vi "Main Page.vi"(8 "error in (no error)":errorcluster, 11 "Node Ptr":T4 format="%.0x") -> (0 "error out":errorcluster)   [LabVIEW 2019, in "Diagnostics Addon System Explorer.lvlib"]
uses:
  Diagnostics Addon System Explorer.lvlib
  <vilib>/NI VeriStand/Custom Device API/Custom Device Item Ref.ctl
  Addon Shared/Types/Protocol.ctl
  Addon Shared/Types/Transport.ctl
  Types/FG.Action.ctl
  <vilib>/NI/NI VeriStand Hardware Resource Discovery/_Types/Filter Type.ctl
  Addon Shared/Types/986x.ctl
  Addon Shared/SubVIs/Constants.vi
  <vilib>/NI VeriStand/Custom Device API/NI VeriStand - Get Item Property.vi
  <vilib>/NI VeriStand/Custom Device API/Get Item Property (Boolean).vi
  <vilib>/NI VeriStand/Custom Device API/Get Item Property (String).vi
  <vilib>/NI VeriStand/Custom Device API/Get Item Property (Dependent File).vi
  <vilib>/NI VeriStand/Custom Device API/Get Item Property (Variant).vi
  <vilib>/NI VeriStand/Custom Device API/Get Item Property (U32).vi
  <vilib>/NI/NI VeriStand Advanced SysDef API/SysDef API/SysDef.Property.Set.vi
  <vilib>/NI/NI VeriStand Advanced SysDef API/_SubVIs/SysDef.Property.Set.String.vi
  <vilib>/NI/NI VeriStand Advanced SysDef API/_SubVIs/SysDef.Property.Set.Variant.vi
  <vilib>/NI/NI VeriStand Advanced SysDef API/_SubVIs/SysDef.Property.Set.U32.vi
  <vilib>/NI/NI VeriStand Advanced SysDef API/_SubVIs/SysDef.Property.Set.Boolean.vi
  <vilib>/NI VeriStand/Custom Device API/Custom Device API.lvlib
  Addon Shared/Diagnostics Addon Shared.lvlib
  <vilib>/NI/NI VeriStand Hardware Resource Discovery/NIVS Hardware Discovery.lvlib
panel:
  in  "Tab Control":T1(tab)
  in  "CAN Browse":bool
  out "Version":string
  in  "Termination":bool
  in  "Name":string
  in  "Description":string
  out "Diagnostic Protocol":T2
  in  "Port":string
  in  "Baud Rate":u64=250000
  in  "Enable Stream":bool
  in  "FD Baud Rate":u64=250000
  in  "Max DLC":u16
  in  "IO Mode":u32(ring) items=["CAN 2.0", "CAN FD", "CAN FD+BRS"]
  in  "Timeout":u32 caption="Comm Timeout (ms)"
  in  "Fill Byte":u8=255 format="%.0x"
  in  "Fill Frame":bool
  in  "Transport Protocol":T3
  in  "VW TP Channel ID":u32 format="%.0x"
  in  "Receive UUDT ID":u32 format="%.0x"
  in  "Receive Extension":u8 format="%.0x"
  in  "Receive ID":u32 format="%.0x"
  in  "Transmit Extension":u8 format="%.0x"
  in  "Transmit ID":u32 format="%.0x"
  in  "NAD":u8
  in  "LIN Cluster":refnum<k21>
  in  "RIO Browse":bool
  in  "RIO Device":string
  in  "Enable Bitfile":bool
  in  "Bitfile Path":path
  in  "Header":cluster{"Section Name":string}={"Section Name"="Custom Device Item Settings"}
  in  "SHDocVw.IWebBrowser":refnum<k7>(container)
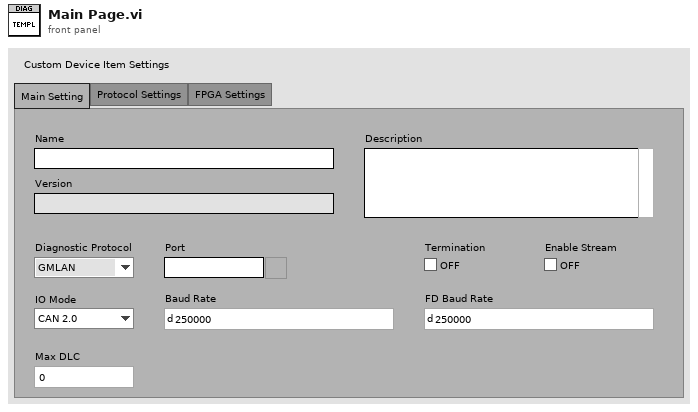
[diagram p1: front panel]
types:
  T1 = enum32{"Main Setting", "Protocol Settings", "FPGA Settings"}
  T2 = typedef "Diagnostics Addon Shared.lvlib/Protocol.ctl" = enum16{"GMLAN", "KWP-2000", "UDS", "User-Defined"}
  T3 = typedef "Diagnostics Addon Shared.lvlib/Transport.ctl" = enum16{"ISO TP - Normal Mode", "ISO TP - Mixed Mode", "VW TP 2.0", "Diagnostics on IP", "ISO TP LIN"}
  T4 = typedef "Custom Device API.lvlib/Custom Device Item Ref.ctl" = u64
  T5 = typedef "Diagnostics Addon System Explorer.lvlib/FG.Action.ctl" = enum16{"Get", "Set"}
  T6 = typedef "Custom Device API.lvlib/Custom Device Item Info.ctl" = cluster{"Name":string, "Is Channel":bool, "GUID":string, "Is Waveform":bool}
  T7 = typedef "Diagnostics Addon Shared.lvlib/986x.ctl" = cluster{"Enable":bool, "RIO Device":string, "Bitfile":path}
  T8 = typedef "Diagnostics Addon Shared.lvlib/CAN.ctl" = cluster{"Interface":T9, "Baud Rate":u64, "Diagnostic Protocol":T2, "Transport Protocol":T3, "Transmit ID":u32, "Receive ID":u32, "Transmit Extension":u8, "Receive Extension":u8, "Receive UUDT ID":u32, "Enable Stream":bool, "VW TP Channel ID":u32, "Fill Frame":bool, "Fill Byte":u8, "Termination":bool, "LIN Cluster":refnum<k21>, "NAD":u8, "IO Mode":u32, "Max DLC":u16, "FD Baud Rate":u64, "Timeout":u32}
  T9 = typedef "Diagnostics Addon Shared.lvlib/CAN.Interface.ctl" = string
  T10 = typedef "NIVS Hardware Discovery.lvlib/Filter Type.ctl" = enum16{"Device Category", "Product Name", "Ethernet", "XNET", "VISA", "FPGA", "EtherCAT Master", "DAQmx", "GPIB", "Serial"}
  T11 = typedef "Custom Device API.lvlib/Custom Device Commands.ctl" = enum16{"Default", "Item renamed", "Shutdown", "Dynamic button pressed"}
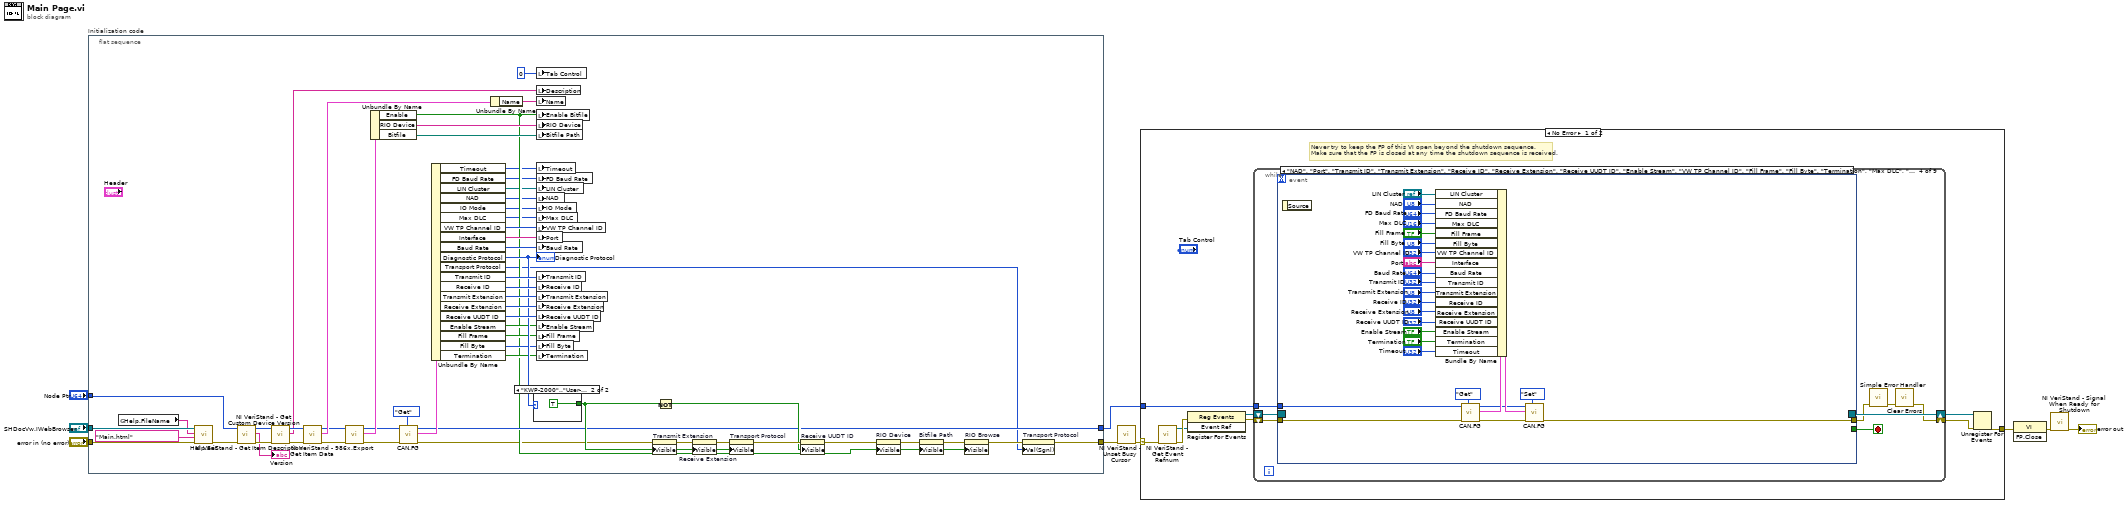
[diagram p0: block diagram]
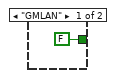
[diagram p2: hidden frame]
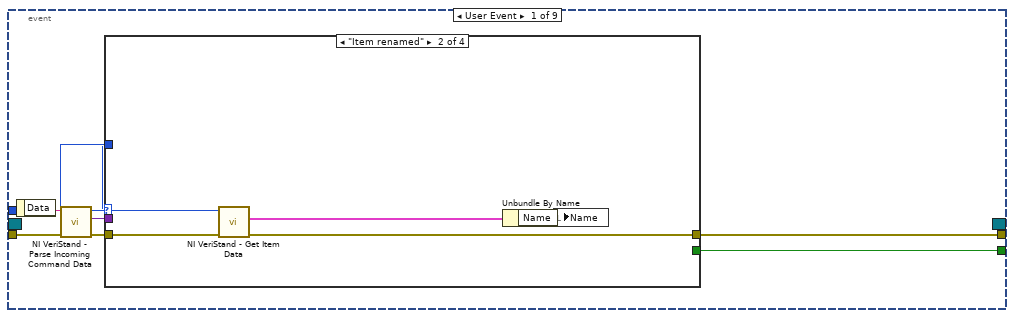
[diagram p3: hidden frame]
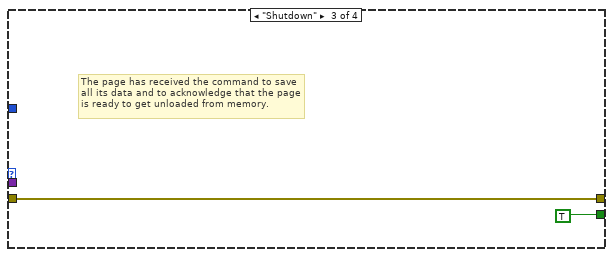
[diagram p5: hidden frame]
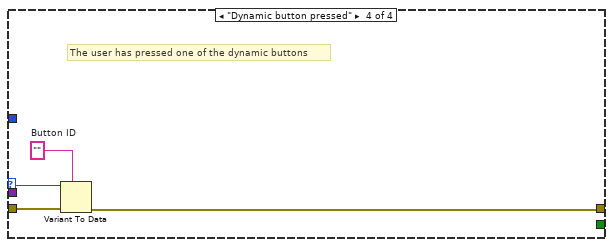
[diagram p6: hidden frame]
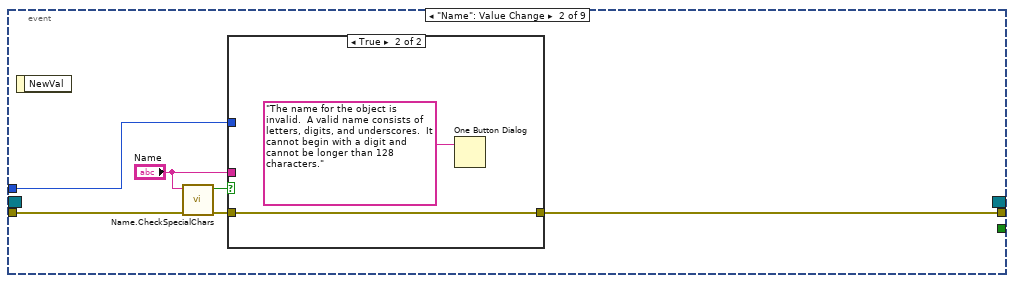
[diagram p7: hidden frame]
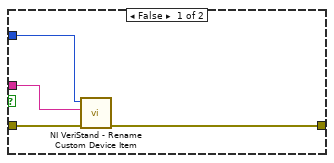
[diagram p8: hidden frame]
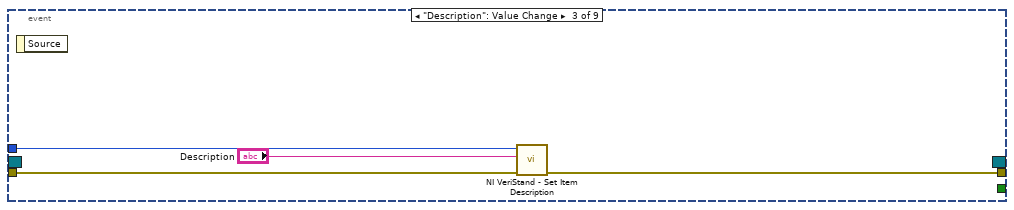
[diagram p9: hidden frame]
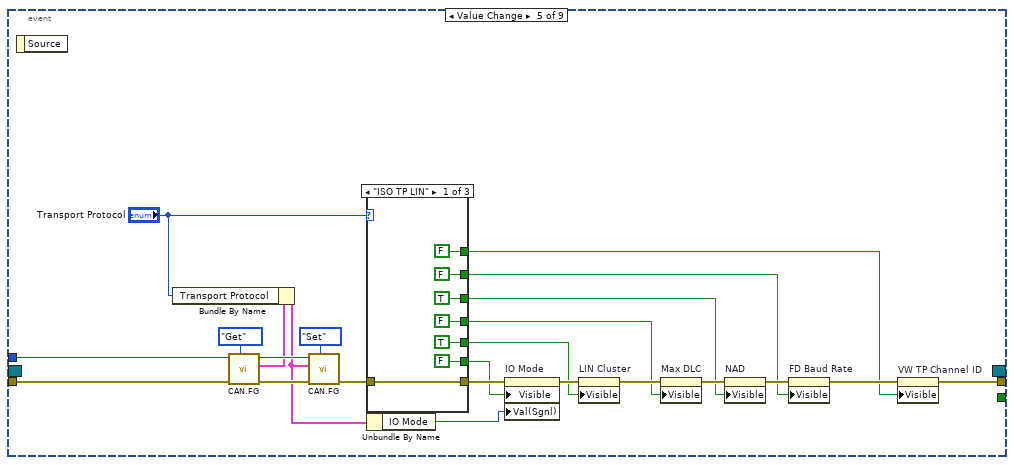
[diagram p10: hidden frame]
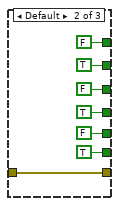
[diagram p11: hidden frame]
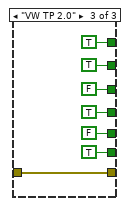
[diagram p12: hidden frame]
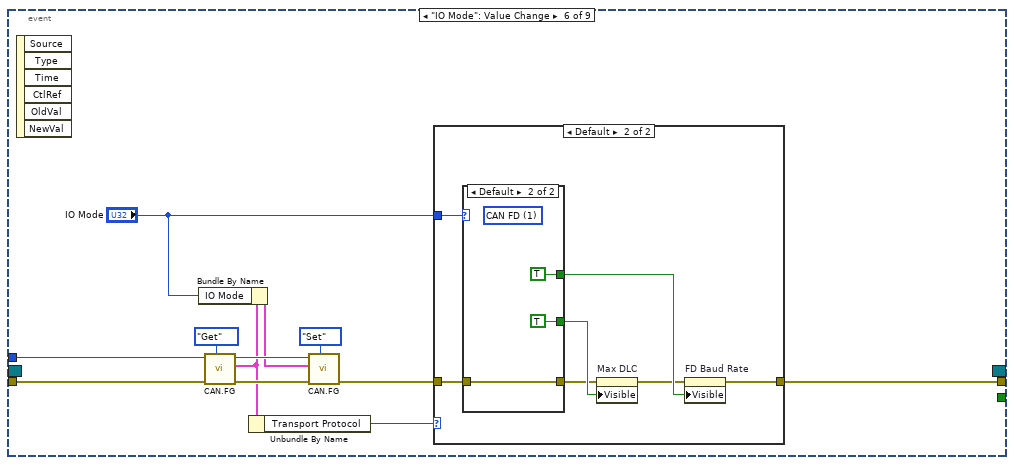
[diagram p13: hidden frame]
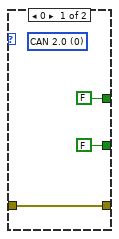
[diagram p15: hidden frame]
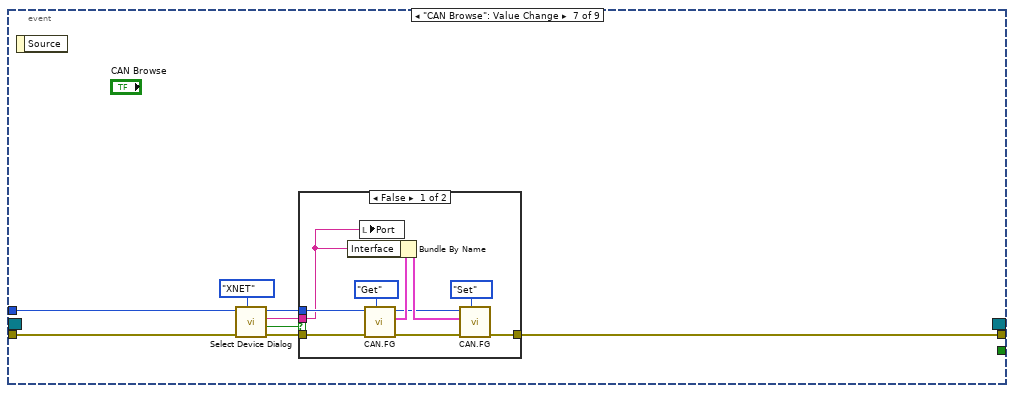
[diagram p16: hidden frame]
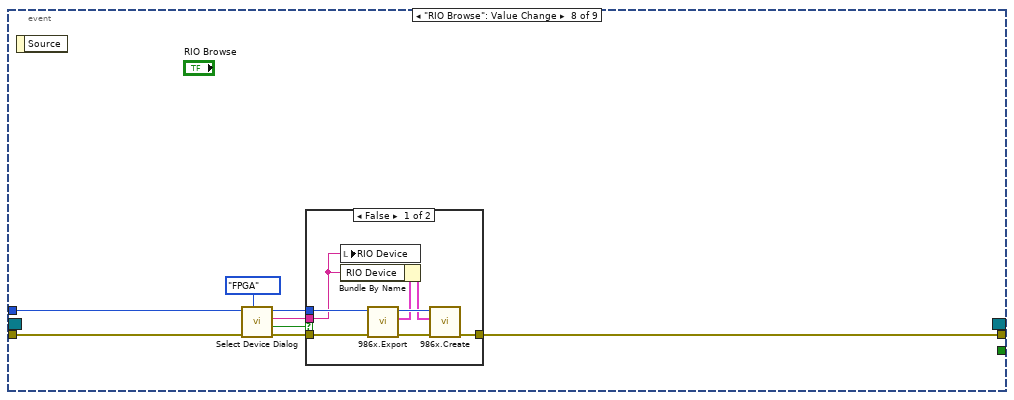
[diagram p18: hidden frame]
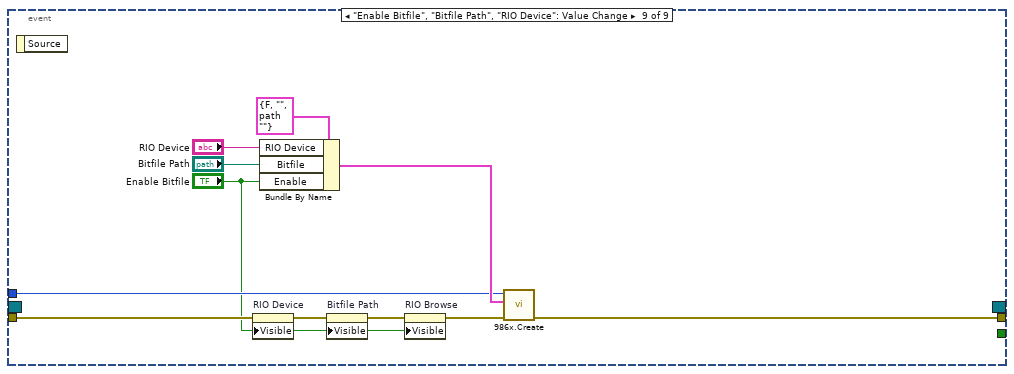
[diagram p20: hidden frame]
diagram:
  n1 = flat-sequence "Initialization code" {
    tunnel: "error in (no error)" -> [w61]
    tunnel: "Node Ptr" -> [w28]
    tunnel: [w11] -> w5
    tunnel: [w30] -> w2
    tunnel: "SHDocVw.IWebBrowser" -> [w60]
    frame #0 {
      n2 = global read "Constants.vi" "Help.FileName"() -> (w10:string)
      n3 = call "Help.Set.vi"("error in (no error)"=w61, "HTML File"="Main.html", "Main CHM File"=w10, "SHDocVw.IWebBrowser2"=w60) -> ("error out"=w29:errorcluster)  [unwired: 7 in]
      n4 = call <vilib>:"NI VeriStand - Get Custom Device Version.vi"("error in (no error)"=w29, "Device Ref in"=w28) -> ("error out"=w26:errorcluster, "Value"=→"Version":string, "Device Ref out"=w27:T4)  [unwired: 7 in]
      n5 = call <vilib>:"NI VeriStand - Get Item Description.vi"("error in (no error)"=w26, "Item Ref in"=w27) -> ("error out"=w64:errorcluster, "Description"=w65:string, "Item Ref out"=w66:T4)  [unwired: 7 out]
      n6 = call <vilib>:"NI VeriStand - Get Item Data.vi"("error in (no error)"=w64, "Item Ref in"=w66) -> ("error out"=w36:errorcluster, "Item Info"=w63:T6, "Item Ref out"=w35:T4)  [unwired: 7 out]
      n7 = call "986x.Export.vi"("error in (no error)"=w36, "Device Item Ref in"=w35) -> ("error out"=w34:errorcluster, "986x Support"=w37:T7, "Item Ref out"=w33:T4)  [unwired: 7 in]
      n8 = Unbundle By Name(w37) -> ("Enable"=w21:bool, "RIO Device"=w31:string, "Bitfile"=w32:path)
      n9 = call "CAN.FG.vi"("Action"=FG.Action."Get", "error in (no error)"=w34, "Device Item Ref in"=w33) -> ("error out"=w13:errorcluster, "Diagnostics Basic Configuration"=w58:T8, "Device Item Ref out"=w30:T4)  [unwired: 6 in]
      n10 = Unbundle By Name(w58) -> ("Timeout"=w12:u32, "FD Baud Rate"=w20:u64, "LIN Cluster"=w16:refnum<k21>, "NAD"=w19:u8, "IO Mode"=w14:u32, "Max DLC"=w18:u16, "VW TP Channel ID"=w44:u32, "Interface"=w57:T9, "Baud Rate"=w56:u64, "Diagnostic Protocol"=w50:T2, "Transport Protocol"=w15:T3, "Transmit ID"=w55:u32, "Receive ID"=w54:u32, "Transmit Extension"=w53:u8, "Receive Extension"=w51:u8, "Receive UUDT ID"=w52:u32, "Enable Stream"=w45:bool, "Fill Frame"=w39:bool, "Fill Byte"=w40:u8, "Termination"=w38:bool)
      "Diagnostic Protocol" <- w50
      n11 = Unbundle By Name(w63) -> ("Name"=w62:string)
      n12 = case shown="\"KWP-2000\"..\"User-Defined\"" w50 {
        tunnel: [FALSE TRUE] -> w42
        frame "GMLAN" {
        }
        frame "KWP-2000".."User-Defined" {
        }
      }
      n13 = local write "Tab Control"(0) -> ()
      n14 = local write "Description"(w65) -> ()
      n15 = local write "Name"(w62) -> ()
      n16 = local write "Enable Bitfile"(w21) -> ()
      n17 = local write "RIO Device"(w31) -> ()
      n18 = local write "Bitfile Path"(w32) -> ()
      n19 = local write "Timeout"(w12) -> ()
      n20 = local write "FD Baud Rate"(w20) -> ()
      n21 = local write "LIN Cluster"(w16) -> ()
      n22 = local write "NAD"(w19) -> ()
      n23 = local write "IO Mode"(w14) -> ()
      n24 = local write "Max DLC"(w18) -> ()
      n25 = local write "VW TP Channel ID"(w44) -> ()
      n26 = local write "Port"(w57) -> ()
      n27 = local write "Baud Rate"(w56) -> ()
      n28 = local write "Transmit ID"(w55) -> ()
      n29 = local write "Receive ID"(w54) -> ()
      n30 = local write "Transmit Extension"(w53) -> ()
      n31 = local write "Receive Extension"(w51) -> ()
      n32 = local write "Receive UUDT ID"(w52) -> ()
      n33 = local write "Enable Stream"(w45) -> ()
      n34 = local write "Fill Frame"(w39) -> ()
      n35 = local write "Fill Byte"(w40) -> ()
      n36 = local write "Termination"(w38) -> ()
      n37 = property on="Transmit Extension" class="DigNum (strict)"(error in=w13, "Visible"=w42) -> (error out=w49:errorcluster)  [unwired: 1 in, 1 out]
      n38 = Not(x=w42) -> (.not. x?=w46:bool)
      n39 = property on="Receive Extension" class="DigNum (strict)"(error in=w49, "Visible"=w42) -> (error out=w48:errorcluster)  [unwired: 1 in, 1 out]
      n40 = property on="Transport Protocol" class="Enum (strict)"(error in=w48, "Visible"=w42) -> (error out=w47:errorcluster)  [unwired: 1 in, 1 out]
      n41 = property on="Receive UUDT ID" class="DigNum (strict)"(error in=w47, "Visible"=w46) -> (error out=w22:errorcluster)  [unwired: 1 in, 1 out]
      n42 = property on="RIO Device" class="Str"(error in=w22, "Visible"=w21) -> (error out=w24:errorcluster)  [unwired: 1 in, 1 out]
      n43 = property on="Bitfile Path" class="Path"(error in=w24, "Visible"=w21) -> (error out=w23:errorcluster)  [unwired: 1 in, 1 out]
      n44 = property on="RIO Browse" class="Bool"(error in=w23, "Visible"=w21) -> (error out=w17:errorcluster)  [unwired: 1 in, 1 out]
      n45 = property on="Transport Protocol" class="Enum (strict)"(error in=w17, "Val(Sgnl)"=w15) -> (error out=w11:errorcluster)  [unwired: 1 in, 1 out]
    }
  }
  n46 = call <vilib>:"NI VeriStand - Unset Busy Cursor.vi"("error in (no error)"=w5) -> ("error out"=w4:errorcluster)  [unwired: 10 out]
  n47 = case shown="No Error" w4 {
    selector: w4 -> [w69 w268]
    tunnel: [w74 w266] -> w9
    tunnel: w2 -> [w70 _]
    frame No Error {
      # "Never try to keep the FP of this VI open beyond the shutdown sequence.\nMake sure that the FP is closed at any time the shutdown sequence is received."
      n48 = call <vilib>:"NI VeriStand - Get Event Refnum.vi"("error in (no error)"=w69) -> ("error out"=w77:errorcluster, "Event Ref"=w73:refnum<user-event>)  [unwired: 9 out]
      n49 = register-events(error in=w77, w73) -> (reference out=w71:refnum<event-registration>, error out=w72:errorcluster)  [unwired: 1 in]
      n50 = while {
        tunnel: w70 -> [w81]
        shift-right: [w78] -> w75
        shift-left: w72 -> [w84]
        shift-right: [w85] -> w76
        shift-left: w71 -> [w83]
        stop <- w82 stop-if-true
        n51 = event shown="[3] \"NAD\", \"Port\", \"Transmit ID\", \"Transmit Extension\", \"Receive ID\", \"Receive Extension\", \"Receive UUDT ID\", \"Enable Stream\", \"VW TP Channel ID\", \"Fill Frame\", \"Fill Byte\", \"Termination\", \"Max DLC\", \"FD Baud Rate\", \"LIN Cluster\", \"Baud Rate\", \"Timeout\": Value Change" {
          selector: w83 -> [_ _ _ _ _ _ _ _ _]
          dyn-events: [_ _ _ _ _ _ _ _ _] -> w85
          timeout: _ -> [_ _ _ _ _ _ _ _ _]
          tunnel: w84 -> [w93 w108 w120 w147 w171 w204 w225 w243 w260]
          tunnel: [w89 _ _ _ _ _ _ _ _] -> w82
          tunnel: [w88 w111 w119 w131 w149 w196 w226 w245 w262] -> w80
          tunnel: w81 -> [w87 w110 w121 w146 w170 w203 w224 w241 w261]
          event User Event {
            n52 = event-data() -> ("Data"=w92:string)  [unwired: 1 out]
            n53 = call <vilib>:"NI VeriStand - Parse Incoming Command Data.vi"("error in (no error)"=w93, "Incoming data"=w92) -> ("error out"=w91:errorcluster, "Outgoing data"=w86:variant, "Action"=w90:T11)  [unwired: 7 out]
            n54 = case shown="\"Item renamed\"" w90 {
              tunnel: w91 -> [w94 w99 w100 w105]
              tunnel: [_ _ TRUE _] -> w89
              tunnel: [w94 w96 w100 w102] -> w88
              tunnel: w87 -> [_ w98 _ _]
              tunnel: w86 -> [_ _ _ w104]
              frame "Default", Default {
              }
              frame "Item renamed" {
                n55 = call <vilib>:"NI VeriStand - Get Item Data.vi"("error in (no error)"=w99, "Item Ref in"=w98) -> ("error out"=w96:errorcluster, "Item Info"=w97:T6)  [unwired: 8 out]
                n56 = Unbundle By Name(w97) -> ("Name"=w95:string)
                n57 = local write "Name"(w95) -> ()
              }
              frame "Shutdown" {
                # "The page has received the command to save all its data and to acknowledge that the page is ready to get unloaded from memory."
              }
              frame "Dynamic button pressed" {
                w103 = ""  # Button ID
                # "The user has pressed one of the dynamic buttons"
                n58 = Variant To Data(error in=w105, type=w103, Variant=w104) -> (error out=w102:errorcluster)  [unwired: 1 out]
              }
            }
          }
          event "Name": Value Change {
            n59 = event-data() -> ()  [unwired: 2 out]
            n60 = call "Name.CheckSpecialChars.vi"("error in"=w108, "Signal Name"="Name") -> ("error out"=w107:errorcluster, "Special Character?"=w106:bool)  [unwired: 8 in]
            n61 = case shown="True" w106 {
              tunnel: [w115 w117] -> w111
              tunnel: w110 -> [w114 _]
              tunnel: "Name" -> [w113 _]
              tunnel: w107 -> [w112 w117]
              frame False {
                n62 = call <vilib>:"NI VeriStand - Rename Custom Device Item.vi"("error in (no error)"=w112, "New Name"=w113, "Item Ref in"=w114) -> ("error out"=w115:errorcluster)  [unwired: 1 in, 7 out]
              }
              frame True {
                n63 = One Button Dialog(message="The name for the object is invalid.  A valid name consists of letters, digits, and underscores.  It cannot begin with a digit and cannot be longer than 128 characters.") -> ()  [unwired: 1 in, 1 out]
              }
            }
          }
          event "Description": Value Change {
            n64 = event-data() -> ()  [unwired: 2 out]
            n65 = call <vilib>:"NI VeriStand - Set Item Description.vi"("error in (no error)"=w120, "Description"="Description", "Item Ref in"=w121) -> ("error out"=w119:errorcluster)  [unwired: 8 out]
          }
          event "NAD", "Port", "Transmit ID", "Transmit Extension", "Receive ID", "Receive Extension", "Receive UUDT ID", "Enable Stream", "VW TP Channel ID", "Fill Frame", "Fill Byte", "Termination", "Max DLC", "FD Baud Rate", "LIN Cluster", "Baud Rate", "Timeout": Value Change {
            n66 = event-data() -> ()  [unwired: 2 out]
            n67 = call "CAN.FG.vi"("Action"=FG.Action."Get", "error in (no error)"=w147, "Device Item Ref in"=w146) -> ("error out"=w133:errorcluster, "Diagnostics Basic Configuration"=w145:T8, "Device Item Ref out"=w132:T4)  [unwired: 6 in]
            n68 = Bundle By Name(cluster=w145, "LIN Cluster"="LIN Cluster", "NAD"="NAD", "FD Baud Rate"="FD Baud Rate", "Max DLC"="Max DLC", "Fill Frame"="Fill Frame", "Fill Byte"="Fill Byte", "VW TP Channel ID"="VW TP Channel ID", "Interface"="Port", "Baud Rate"="Baud Rate", "Transmit ID"="Transmit ID", "Transmit Extension"="Transmit Extension", "Receive ID"="Receive ID", "Receive Extension"="Receive Extension", "Receive UUDT ID"="Receive UUDT ID", "Enable Stream"="Enable Stream", "Termination"="Termination", "Timeout"="Timeout") -> (w134:T8)
            n69 = call "CAN.FG.vi"("Action"=FG.Action."Set", "error in (no error)"=w133, "Diagnostics Basic Configuration"=w134, "Device Item Ref in"=w132) -> ("error out"=w131:errorcluster)  [unwired: 5 in, 2 out]
          }
          event Value Change {
            n70 = event-data() -> ()  [unwired: 2 out]
            n71 = call "CAN.FG.vi"("Action"=FG.Action."Get", "error in (no error)"=w171, "Device Item Ref in"=w170) -> ("error out"=w168:errorcluster, "Diagnostics Basic Configuration"=w165:T8, "Device Item Ref out"=w167:T4)  [unwired: 6 in]
            n72 = Bundle By Name(cluster=w165, "Transport Protocol"="Transport Protocol") -> (w152:T8)
            n73 = call "CAN.FG.vi"("Action"=FG.Action."Set", "error in (no error)"=w168, "Diagnostics Basic Configuration"=w152, "Device Item Ref in"=w167) -> ("error out"=w163:errorcluster)  [unwired: 5 in, 2 out]
            n74 = case shown="\"ISO TP LIN\"" "Transport Protocol" {
              tunnel: w163 -> [w178 w185 w192]
              tunnel: [w178 w185 w192] -> w158
              tunnel: [FALSE ("Visible") TRUE ("Visible") TRUE ("Visible")] -> w157
              tunnel: [TRUE ("Visible") FALSE ("Visible") FALSE ("Visible")] -> w156
              tunnel: [FALSE ("Visible") TRUE ("Visible") TRUE ("Visible")] -> w155
              tunnel: [TRUE ("Visible") FALSE ("Visible") FALSE ("Visible")] -> w154
              tunnel: [FALSE ("Visible") TRUE ("Visible") TRUE ("Visible")] -> w153
              tunnel: [FALSE ("Visible") FALSE ("Visible") TRUE ("Visible")] -> w148
              frame "ISO TP LIN" {
              }
              frame Default {
              }
              frame "VW TP 2.0" {
              }
            }
            n75 = Unbundle By Name(w152) -> ("IO Mode"=w151:u32)
            n76 = property on="IO Mode" class="Ring (strict)"(error in=w158, "Visible"=w157, "Val(Sgnl)"=w151) -> (error out=w160:errorcluster)  [unwired: 1 in, 1 out]
            n77 = property on="LIN Cluster" class="XNET (strict)"(error in=w160, "Visible"=w156) -> (error out=w159:errorcluster)  [unwired: 1 in, 1 out]
            n78 = property on="Max DLC" class="DigNum (strict)"(error in=w159, "Visible"=w155) -> (error out=w161:errorcluster)  [unwired: 1 in, 1 out]
            n79 = property on="NAD" class="DigNum (strict)"(error in=w161, "Visible"=w154) -> (error out=w162:errorcluster)  [unwired: 1 in, 1 out]
            n80 = property on="FD Baud Rate" class="DigNum (strict)"(error in=w162, "Visible"=w153) -> (error out=w150:errorcluster)  [unwired: 1 in, 1 out]
            n81 = property on="VW TP Channel ID" class="DigNum (strict)"(error in=w150, "Visible"=w148) -> (error out=w149:errorcluster)  [unwired: 1 in, 1 out]
          }
          event "IO Mode": Value Change {
            n82 = event-data() -> ()  [unwired: 7 out]
            n83 = call "CAN.FG.vi"("Action"=FG.Action."Get", "error in (no error)"=w204, "Device Item Ref in"=w203) -> ("error out"=w201:errorcluster, "Diagnostics Basic Configuration"=w194:T8, "Device Item Ref out"=w200:T4)  [unwired: 6 in]
            n84 = Bundle By Name(cluster=w194, "IO Mode"="IO Mode") -> (w198:T8)
            n85 = Unbundle By Name(w194) -> ("Transport Protocol"=w193:T3)
            n86 = call "CAN.FG.vi"("Action"=FG.Action."Set", "error in (no error)"=w201, "Diagnostics Basic Configuration"=w198, "Device Item Ref in"=w200) -> ("error out"=w197:errorcluster)  [unwired: 5 in, 2 out]
            n87 = case shown="Default" w193 {
              tunnel: w197 -> [w205 w212]
              tunnel: [w205 w211] -> w196
              tunnel: "IO Mode" -> [_ w208]
              frame "ISO TP LIN" {
              }
              frame Default {
                n88 = case shown="Default" w208 {
                  tunnel: w212 -> [w215 w218]
                  tunnel: [w215 w218] -> w207
                  tunnel: [FALSE ("Visible") TRUE ("Visible")] -> w210
                  tunnel: [FALSE ("Visible") TRUE ("Visible")] -> w209
                  frame 0 {
                    (unwired) u32 0 items=["CAN 2.0", "CAN FD", "CAN FD+BRS"] ("IO Mode")
                  }
                  frame Default {
                    (unwired) u32 1 items=["CAN 2.0", "CAN FD", "CAN FD+BRS"] ("IO Mode")
                  }
                }
                n89 = property on="Max DLC" class="DigNum (strict)"(error in=w207, "Visible"=w210) -> (error out=w206:errorcluster)  [unwired: 1 in, 1 out]
                n90 = property on="FD Baud Rate" class="DigNum (strict)"(error in=w206, "Visible"=w209) -> (error out=w211:errorcluster)  [unwired: 1 in, 1 out]
              }
            }
          }
          event "CAN Browse": Value Change {
            n91 = event-data() -> ()  [unwired: 2 out]
            n92 = call <vilib>:"Select Device Dialog.vi"("Filter Type"=Filter_Type."XNET", "error in (no error)"=w225, "Item Ref in"=w224) -> ("error out"=w222:errorcluster, "Cancelled?"=w219:bool, "Selected Alias"=w220:string, "Item Ref out"=w223:T4)  [unwired: 5 in]
            n93 = case shown="False" w219 {
              tunnel: [w231 w237] -> w226
              tunnel: w223 -> [w229 _]
              tunnel: w222 -> [w228 w237]
              tunnel: w220 -> [w227 _]
              frame False {
                n94 = local write "Port"(w227) -> ()
                n95 = call "CAN.FG.vi"("Action"=FG.Action."Get", "error in (no error)"=w228, "Device Item Ref in"=w229) -> ("error out"=w233:errorcluster, "Diagnostics Basic Configuration"=w236:T8, "Device Item Ref out"=w232:T4)  [unwired: 6 in]
                n96 = Bundle By Name(cluster=w236, "Interface"=w227) -> (w234:T8)
                n97 = call "CAN.FG.vi"("Action"=FG.Action."Set", "error in (no error)"=w233, "Diagnostics Basic Configuration"=w234, "Device Item Ref in"=w232) -> ("error out"=w231:errorcluster)  [unwired: 5 in, 2 out]
              }
              frame True {
              }
            }
          }
          event "RIO Browse": Value Change {
            n98 = event-data() -> ()  [unwired: 2 out]
            n99 = call <vilib>:"Select Device Dialog.vi"("Filter Type"=Filter_Type."FPGA", "error in (no error)"=w243, "Item Ref in"=w241) -> ("error out"=w242:errorcluster, "Cancelled?"=w238:bool, "Selected Alias"=w239:string, "Item Ref out"=w240:T4)  [unwired: 5 in]
            n100 = case shown="False" w238 {
              tunnel: [w253 w254] -> w245
              tunnel: w242 -> [w248 w254]
              tunnel: w240 -> [w247 _]
              tunnel: w239 -> [w246 _]
              frame False {
                n101 = local write "RIO Device"(w246) -> ()
                n102 = call "986x.Export.vi"("error in (no error)"=w248, "Device Item Ref in"=w247) -> ("error out"=w252:errorcluster, "986x Support"=w250:T7, "Item Ref out"=w251:T4)  [unwired: 7 in]
                n103 = Bundle By Name(cluster=w250, "RIO Device"=w246) -> (w249:T7)
                n104 = call "986x.Create.vi"("error in (no error)"=w252, "986x Support"=w249, "Device Item Ref in"=w251) -> ("error out"=w253:errorcluster)  [unwired: 7 in, 1 out]
              }
              frame True {
              }
            }
          }
          event "Enable Bitfile", "Bitfile Path", "RIO Device": Value Change {
            n105 = event-data() -> ()  [unwired: 2 out]
            n106 = property on="RIO Device" class="Str"(error in=w260, "Visible"="Enable Bitfile") -> (error out=w259:errorcluster)  [unwired: 1 in, 1 out]
            n107 = Bundle By Name(cluster=T7 {"Enable"=FALSE, "RIO Device"="", "Bitfile"=path ""} ("986x Support"), "RIO Device"="RIO Device", "Bitfile"="Bitfile Path", "Enable"="Enable Bitfile") -> (w263:T7)
            n108 = property on="Bitfile Path" class="Path"(error in=w259, "Visible"="Enable Bitfile") -> (error out=w257:errorcluster)  [unwired: 1 in, 1 out]
            n109 = property on="RIO Browse" class="Bool"(error in=w257, "Visible"="Enable Bitfile") -> (error out=w256:errorcluster)  [unwired: 1 in, 1 out]
            n110 = call "986x.Create.vi"("error in (no error)"=w256, "986x Support"=w263, "Device Item Ref in"=w261) -> ("error out"=w262:errorcluster)  [unwired: 7 in, 1 out]
          }
        }
        n111 = call <vilib>:"Simple Error Handler.vi"("error in (no error)"=w80) -> ("error out"=w79:errorcluster)  [unwired: 1 in, 7 out]
        n112 = call <vilib>:"Clear Errors.vi"("error in (no error)"=w79) -> ("error out"=w78:errorcluster)  [unwired: 1 in, 5 out]
      }
      n113 = Unregister For Events(event registration refnum=w76, error in=w75) -> (error out=w74:errorcluster)
    }
    frame Error {
      n114 = call <vilib>:"Simple Error Handler.vi"("error in (no error)"=w268) -> ("error out"=w267:errorcluster)  [unwired: 1 in, 7 out]
      n115 = call <vilib>:"Clear Errors.vi"("error in (no error)"=w267) -> ("error out"=w266:errorcluster)  [unwired: 1 in, 5 out]
    }
  }
  n116 = invoke class="VI" method="FP.Close"(error in=w9) -> (error out=w8:errorcluster)  [unwired: 2 in, 2 out]
  n117 = call <vilib>:"NI VeriStand - Signal When Ready for Shutdown.vi"("error in (no error)"=w8) -> ("error out"=→"error out":errorcluster)  [unwired: 10 out]
